vi "SetUIAvailability.vi"(8 "error in (no error)":errorcluster, 10 "Has UI?(T)":bool, 11 "Analyser in":refnum<class "Analyser.lvclass">) -> (0 "error out":errorcluster, 3 "Analyser out":refnum<class "Analyser.lvclass">)   [LabVIEW 2020, in "Analyser.lvlib" / "Analyser.lvclass"]
uses:
  Analyser.lvclass
  Analyser.lvclass/Analyser.ctl
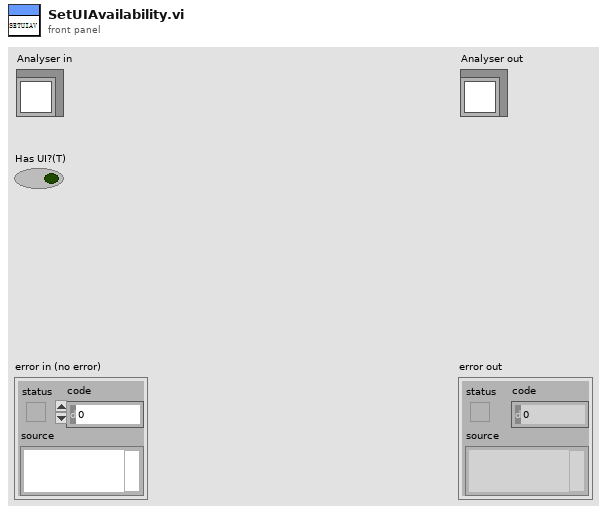
[diagram p1: front panel]
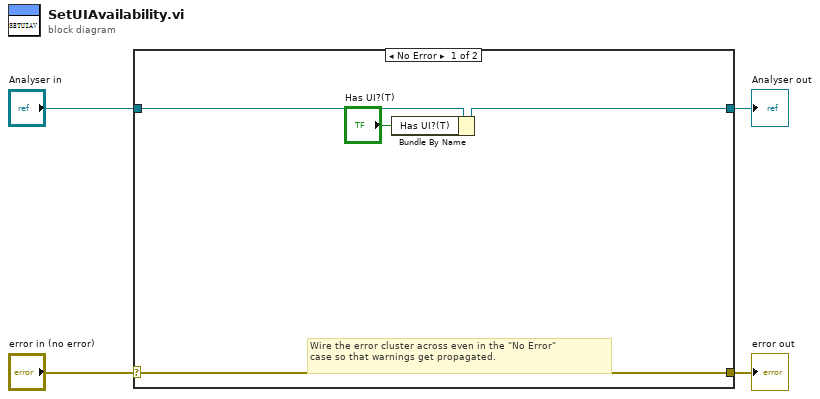
[diagram p0: block diagram]
diagram:
  n1 = case shown="No Error" "error in (no error)" {
    selector: "error in (no error)" -> [w7 w10]
    tunnel: [w7 w10] -> w3
    tunnel: [w6 w9] -> w1
    tunnel: "Analyser in" -> [w8 w9]
    frame No Error {
      # "Wire the error cluster across even in the \"No Error\"\ncase so that warnings get propagated."
      n2 = Bundle By Name(cluster=w8, "Has UI?(T)"="Has UI?(T)") -> (w6:refnum<class "Analyser.lvclass">)
    }
    frame Error {
    }
  }
  "error out" <- w3
  "Analyser out" <- w1
